vi "ReadAsPixmapCore.vi"(4 "mask":u8[](array[numeric]), 5 "Pixel Formats":T2, 6 "colours":u32[](array[numeric]), 7 "Top Left Point":T3, 8 "error in (no error)":errorcluster, 11 "Buffer In":refnum<class "Buffer.lvclass">) -> (0 "error out":errorcluster, 3 "pixmap":T1)   [LabVIEW 2020, in "Buffer.lvclass"]
uses:
  Buffer.lvclass
  Buffer.lvclass/Buffer.ctl
  <vilib>/picture/picture.llb/imagedata.ctl
  bin/gindustrialcam_32-1.dll
  Picture Top Left Point Offset.ctl
  Pixel Formats.ctl
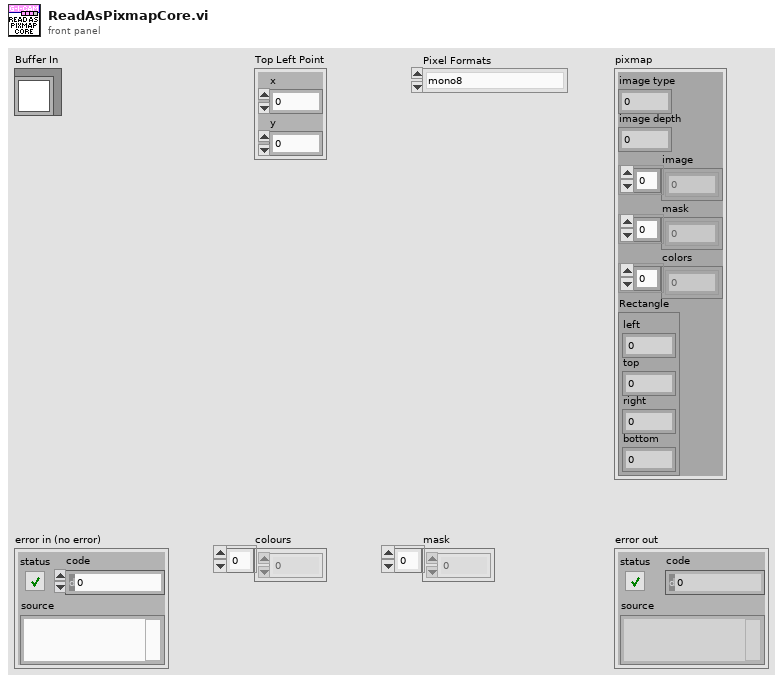
[diagram p1: front panel]
types:
  T1 = typedef "imagedata.ctl" = cluster{"image type":i32, "image depth":i32, "image":u8[], "mask":u8[], "colors":u32[], "Rectangle":cluster{"left":i16, "top":i16, "right":i16, "bottom":i16}}
  T2 = typedef "Buffer.lvclass/Pixel Formats.ctl" = enum16{"mono8", "mono10", "mono10p", "mono12", "mono12p", "mono14", "mono14p", "mono16", "RGB8", "BGR8"}
  T3 = typedef "Buffer.lvclass/Picture Top Left Point Offset.ctl" = cluster{"x":i16, "y":i16}
  T4 = cluster{"op_code":i16, "length":i32, "image_bytes_length":i32, "top":i16, "left":i16, "bottom":i16, "right":i16, "bitwidth":i16, "foreground":u32, "background":u32}
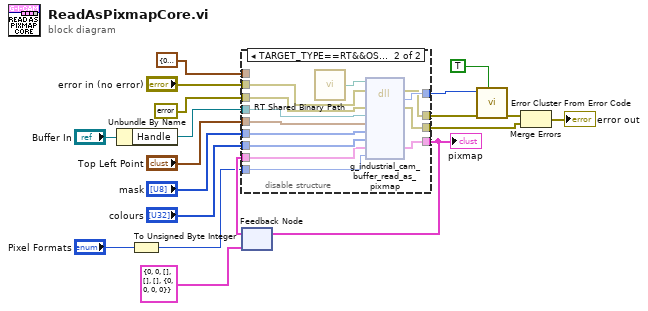
[diagram p0: block diagram]
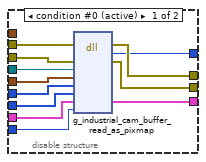
[diagram p2: hidden frame]
diagram:
  n1 = Unbundle By Name("Buffer In") -> ("Handle"=w4:refnum<data-value>)
  n2 = To Unsigned Byte Integer(number="Pixel Formats") -> (unsigned 8bit integer=w5:u8)
  n3 = feedback #1(T1 {"image type"=0, "image depth"=0, "image"=[], "mask"=[], "colors"=[], "Rectangle"={"left"=0, "top"=0, "right"=0, "bottom"=0}} ("image data")) -> (w8:T1)
  n4 = disable-structure shown="TARGET_TYPE==RT&&OS==Linux" {
    disable-tunnel: "Top Left Point" -> [w31 w40]
    disable-tunnel: "error in (no error)" -> [w30 w43]
    disable-tunnel: errorcluster {"status"=FALSE, "code"=0, "source"=""} ("error constant") -> [w29 w42]
    disable-tunnel: T4 {"op_code"=0, "length"=0, "image_bytes_length"=0, "top"=0, "left"=0, "bottom"=0, "right"=0, "bitwidth"=0, "foreground"=0, "background"=0} -> [_ _]
    disable-tunnel: [w28 w33] -> w12
    disable-tunnel: [w27 w35] -> w11
    disable-tunnel: [w26 w32] -> w10
    disable-tunnel: [w25 w34] -> w9
    disable-tunnel: w8 -> [w22 w37]
    disable-tunnel: w5 -> [w24 w36]
    disable-tunnel: w4 -> [w23 w41]
    disable-tunnel: "mask" -> [w21 w39]
    disable-tunnel: "colours" -> [w20 w38]
    frame condition #0 (active) {
      n5 = dll-call lib="C:/serenial/lib/g-industrial-camera/LabVIEW/g_industrial_cam/bin/gindustrialcam_*-1.*" fn="g_industrial_cam_buffer_read_as_pixmap" ("g_ar_toolkit.*.*:g_ar_tk_image_draw_picture")(error in=w30, "error_cluster"=w29, "EDVR src"=w23, "top_left"=w31, "mask"=w21, "colours"=w20, "pixmap"=w22, "pixel_format"=w24) -> (error out=w28:errorcluster, "return type"=w27:i32, "error_cluster"=w26:errorcluster, "pixmap"=w25:T1)  [unwired: 7 in, 1 out]
    }
    frame condition #1 {
      n6 = call "RT Shared Binary Path.vi"() -> ("Path"=w44:path)
      n7 = dll-call lib="?" fn="g_industrial_cam_buffer_read_as_pixmap" ("g_ar_toolkit.*.*:g_ar_tk_image_draw_picture")(path in=w44, error in=w43, "error_cluster"=w42, "EDVR src"=w41, "top_left"=w40, "mask"=w39, "colours"=w38, "pixmap"=w37, "pixel_format"=w36) -> (error out=w33:errorcluster, "return type"=w35:i32, "error_cluster"=w32:errorcluster, "pixmap"=w34:T1)  [unwired: 6 in, 1 out]
    }
  }
  "pixmap" <- w9
  n8 = feedback-in #1(w9) -> ()
  n9 = call <vilib>:"Error Cluster From Error Code.vi"("show call chain? (False)"=TRUE, "error in (no error)"=w12, "error code (0)"=w11) -> ("error out"=w18:errorcluster)  [unwired: 6 in]
  n10 = Merge Errors(w18, w10) -> (→"error out":errorcluster)
